vi "Set VDD Voltage and MeasV_Module.vi"(7 "Publishable ID":string="PreFuse_Vio_Meas", 8 "error in (no error)":errorcluster, 9 "VDD voltage level":dbl=1.8 caption="voltage level" format="%_6p", 10 "Pins":string[](array[string])=["VDD"], 11 "Semiconductor Module Context":T1) -> (0 "error out":errorcluster, 2 "Instrument Sessions Out":refnum<k15>[](array[refnum]), 3 "Semiconductor Module Context Out":T1)   [LabVIEW 2013]
uses:
  <vilib>/NI_TestStand_SemiconductorModule/NI_TestStand_Semiconductor_Module.lvlibp/PinMap/General/SemiconductorModuleContext.ctl
  <vilib>/NI_TestStand_SemiconductorModule/NI_TestStand_Semiconductor_Module.lvlibp/PinMap/DC Power/PinsToNIDCPowerSessions.vi
  <vilib>/NI_TestStand_SemiconductorModule/NI_TestStand_Semiconductor_Module.lvlibp/PinMap/Deprecated/PublishDataDoubleSinglePinSingleInstrument.vi
  <vilib>/NI_TestStand_SemiconductorModule/NI_TestStand_Semiconductor_Module.lvlibp
panel:
  out "voltage measurements":dbl[][](array[numeric])
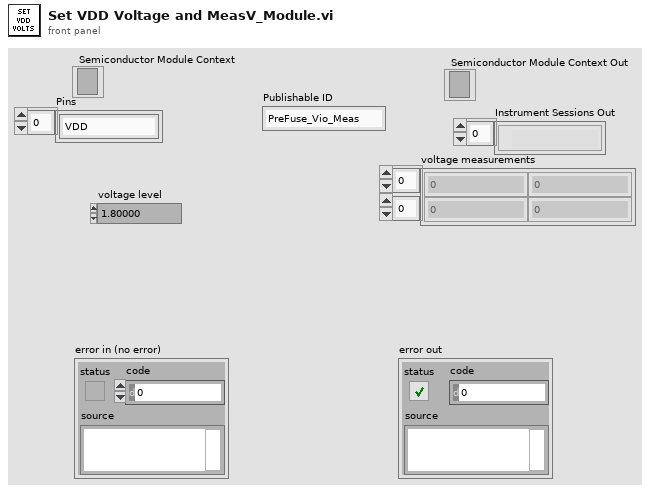
[diagram p1: front panel]
types:
  T1 = typedef "NI_TestStand_Semiconductor_Module.lvlibp/SemiconductorModuleContext.ctl" = refnum<k7>
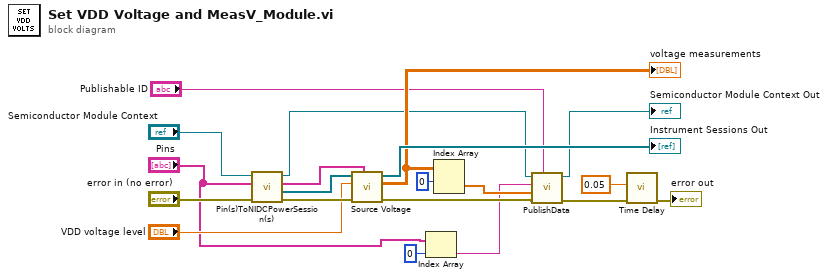
[diagram p0: block diagram]
diagram:
  n1 = call-poly <vilib>:"Pin(s)ToNIDCPowerSession(s).vi"("error in (no error)"="error in (no error)", "Pins"="Pins", "Semiconductor Module Context"="Semiconductor Module Context") -> ("error out"=w18:errorcluster, "Instrument Sessions"=w17:refnum<k15>[], "Channel Lists"=w4:string[], "Semiconductor Module Context Out"=w10:T1)  [unwired: 4 in, 1 out]
  n2 = call "Source Voltage.vi"("Channel Lists"=w4, "error in (no error)"=w18, "voltage level"="VDD voltage level", "Instrument Sessions In"=w17) -> ("error out"=w12:errorcluster, "voltage measurements"=w14:dbl[][], "Instrument Sessions Out"=→"Instrument Sessions Out":refnum<k15>[])  [unwired: 4 in, 1 out]
  "voltage measurements" <- w14
  n3 = Index Array(array="Pins", index=0) -> (element=w2:string)
  n4 = Index Array(array=w14, index (row)=0) -> (element=w8:dbl[])  [unwired: 1 in]
  n5 = call-poly <vilib>:"PublishData.vi"("Measurement Id"="Publishable ID", "error in (no error)"=w12, "Data In"=w8, "Pin"=w2, "Semiconductor Module Context"=w10) -> ("error out"=w7:errorcluster, "Semiconductor Module Context Out"=→"Semiconductor Module Context Out":T1)  [unwired: 5 in]
  n6 = call "Time Delay"("error in (no error)"=w7, "Delay Time (s)"=0.05) -> ("error out"=→"error out":errorcluster)  [unwired: 9 in]
